vi "Read_Flow_Press_Bkgd_Mvg_avg.vi"() -> ()   [LabVIEW 2016]
uses:
  <userlib>/Fluigent/Fluigent MFCS/FluigentMFCS_Full.llb/MFCS_EZ Detect.vi
  <userlib>/Fluigent/Fluigent MFCS/FluigentMFCS_Full.llb/MFCS_EZ Initialization.vi
  Globals/PressuresGlobal.vi
  <vilib>/Analysis/baseanly.llb/Unimode.vi
  <vilib>/imath/engines/lvmath2/RunTimeEngine/BuiltInFunctions/size/NIMS_I32=size(GM,I32).vi
  <instcachedir>/0/NIMS_I32=size(GM,I32)_9B6975FE2A37478D9DF1A6A9597B9E6B.lvgen/NIMS_I32=size(GM,I32)_9B6975FE2A37478D9DF1A6A9597B9E6B_004.vi
  <vilib>/imath/engines/lvmath2/RunTimeEngine/BuiltInFunctions/zeros/NIMS_V=zeros(I32,I32).vi
  <vilib>/imath/engines/lvmath2/RunTimeEngine/ErrorHandling/NIMS_Create Error From Enums.vi
  <vilib>/imathl/engines/lvmath/Functions/Error Handling/Create Error.vi
  <vilib>/imath/engines/lvmath2/RunTimeEngine/RangeToken/NIMS_Range_R2 - Integer.vi
  <instcachedir>/0/NIMS_Range_R2 - Integer_416A044C4F024DBE8E97DA138CB3186F.lvgen/NIMS_Range_R2 - Integer_416A044C4F024DBE8E97DA138CB3186F_000.vi
  <vilib>/imath/engines/lvmath2/RunTimeEngine/CommandStatement/MC_CommandStatement_break.vi
  <vilib>/imath/engines/lvmath2/RunTimeEngine/IndexRead/NIMS M($,S).vi
  <instcachedir>/0/NIMS M($,S)_3E5749BBB62E49528D4765A77F1F6D98.lvgen/NIMS M($,S)_3E5749BBB62E49528D4765A77F1F6D98_000.vi
  <vilib>/imath/engines/lvmath2/RunTimeEngine/BuiltInFunctions/sets_unique/NIMS_sets_unique(GV).vi
  <instcachedir>/0/NIMS_sets_unique(GV)_BC60CBD939E647F382369330BF9EA64D.lvgen/NIMS_sets_unique(GV)_BC60CBD939E647F382369330BF9EA64D_001.vi
  <vilib>/imath/engines/lvmath2/RunTimeEngine/BuiltInFunctions/length/NIMS_length(GV).vi
  <instcachedir>/0/NIMS_length(GV)_08A3D13377FD4E4B96F5795FBF3698FA.lvgen/NIMS_length(GV)_08A3D13377FD4E4B96F5795FBF3698FA_000.vi
  <vilib>/imath/engines/lvmath2/RunTimeEngine/IndexReplace/NIMS V(S)=S.vi
  <instcachedir>/0/NIMS V(S)=S_5B9D821375184D3582A2146CD1A04ED7.lvgen/NIMS V(S)=S_5B9D821375184D3582A2146CD1A04ED7_003.vi
  <vilib>/imath/engines/lvmath2/RunTimeEngine/NodeEndStatement/NIMS_NodeEndStatement_Output.vi
  <instcachedir>/0/NIMS_NodeEndStatement_Output_53EC0D466D134D7ABD903AC30B43404B.lvgen/NIMS_NodeEndStatement_Output_53EC0D466D134D7ABD903AC30B43404B_004.vi
  <vilib>/imath/engines/lvmath2/RunTimeEngine/ErrorHandling/NIMS_Finalize Error.vi
  <userlib>/Fluigent/Fluigent MFCS/FluigentMFCS_Full.llb/MFCS_EZ Read All Channels Pressure.vi
  <vilib>/Analysis/NI_AALBase.lvlib
panel:
  in  "reset averaging":bool
  out "Pressure Stable?":bool=TRUE
  in  "reset volume":bool
  out "Volume":dbl[](array[numeric])
  out "Median":dbl[](array[numeric])
  out "Mode":dbl[](array[numeric])
  out "numUnique":i32[](array[numeric])
  out "sum":dbl
  out "pressure array":dbl[][](array[numeric])
  in  "Time to include":dbl=5.0
  out "dt(calc)":dbl
  out "freq (Hz)":dbl
  out "Sample Rate":dbl(graph)
  in  "stop":bool
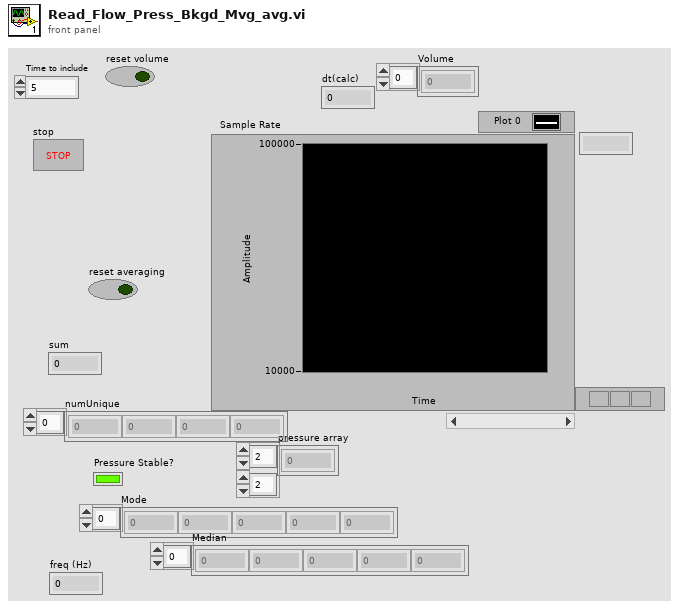
[diagram p1: front panel]
types:
  T1 = cluster{"Time":dbl, "All Flow-Rates":dbl[], "Flow 2 Filter Time":dbl, "Flow 1 Filter Time":dbl}
  T2 = typedef "_EZmfcsSN.ctl" = u16
  T3 = typedef "_EZmfcsRefNum.ctl" = refnum<k1>
  T4 = typedef "_frpRefNum" = refnum<k1>
  T5 = cluster{"relative seconds":dbl, "All Flow-Rates":dbl[], "Flow 1 Filter Time":dbl, "Flow 2 Filter Time":dbl}
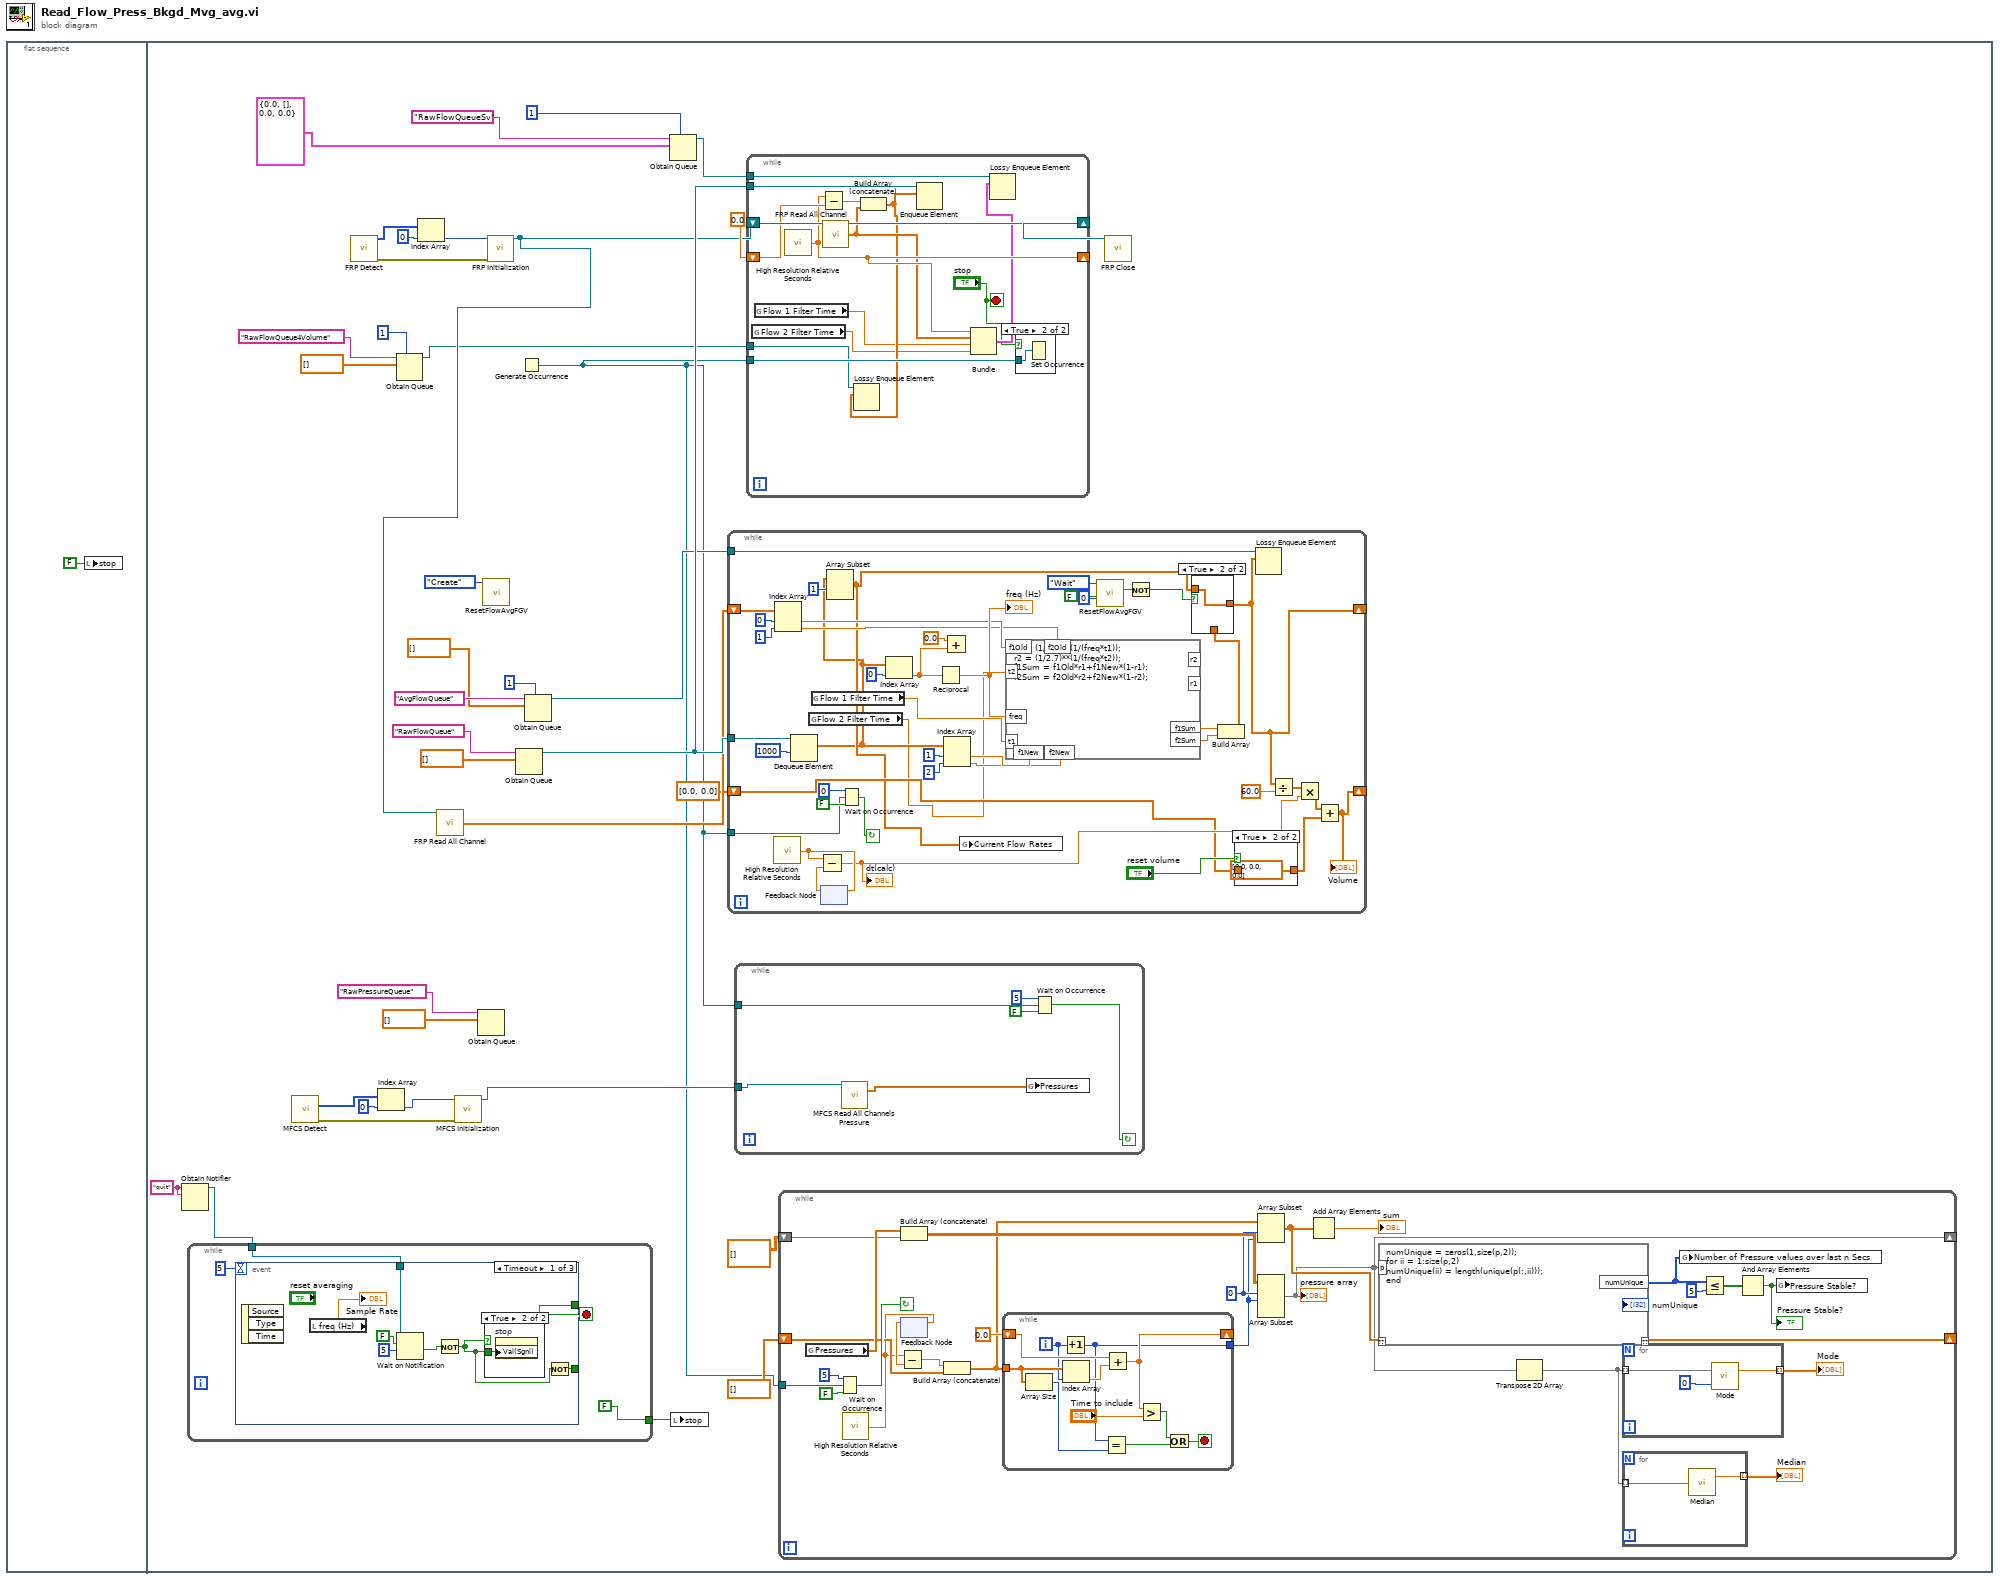
[diagram p0: block diagram]
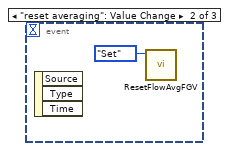
[diagram p5: hidden frame]
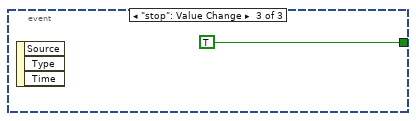
[diagram p6: hidden frame]
diagram:
  n1 = flat-sequence {
    frame #0 {
      n2 = local write "stop"(FALSE ("stop")) -> ()
    }
    frame #1 {
      w5 = "quit" ("name (unnamed)")
      n3 = Obtain Notifier(name (unnamed)=w5, notification data type=w5) -> (notifier out=w3:refnum<notifier>)  [unwired: 2 in, 2 out]
      n4 = while {
        tunnel: w3 -> [w247]
        tunnel: [FALSE] -> w2
        stop <- w248 stop-if-true
        n5 = event shown="[0] Timeout" {
          selector: _ -> [_ _ _]
          dyn-events: _ -> [_ _ _]
          timeout: 5 -> [_ _ _]
          tunnel: [_ _ TRUE] -> w248
          tunnel: w247 -> [w252 _ _]
          tunnel: [w250 _ _] -> _
          event Timeout {
            n6 = event-data() -> ()  [unwired: 1 in, 3 out]
            n7 = local read "freq (Hz)"() -> (→"Sample Rate":dbl)
            n8 = Wait on Notification(notifier=w252, ignore previous (F)=FALSE, timeout in ms (-1)=5) -> (timed out?=w254:bool)  [unwired: 1 in, 3 out]
            n9 = Not(x=w254) -> (.not. x?=w251:bool)
            n10 = case shown="True" w251 {
              tunnel: w251 -> [_ w257]
              frame False {
              }
              frame True {
                n11 = property on="stop" class="Bool (strict)"("Val(Sgnl)"=w257) -> ()  [unwired: 2 in, 2 out]
              }
            }
            n12 = Not(x=w251) -> (.not. x?=w250:bool)
          }
          event "reset averaging": Value Change {
            n13 = event-data() -> ()  [unwired: 1 in, 3 out]
            n14 = call "ResetFlowAvgFGV.vi"("Action"=enum16{"Create", "Set", "Wait"}."Set") -> ()  [unwired: 10 in, 1 out]
          }
          event "stop": Value Change {
            n15 = event-data() -> ()  [unwired: 1 in, 3 out]
          }
        }
      }
      n16 = call-poly <userlib>:"MFCS Detect.vi"() -> ("[SN MFCS_EZ]"=w15:T2[], "error out"=w17:errorcluster)  [unwired: 14 in]
      n17 = call <userlib>:"FRP Detect.vi"() -> ("FLOWBOARD List"=w39:u16[], "error out"=w37:errorcluster)  [unwired: 14 in]
      n18 = Index Array(array=w15, index=0) -> (element=w16:T2)
      n19 = Obtain Queue(max queue size (-1, unlimited)=1, name (unnamed)="RawFlowQueue4Volume", element data type=dbl[] [] ("appended array")) -> (queue out=w7:refnum<queue>)  [unwired: 2 in, 2 out]
      n20 = Index Array(array=w39, index=0) -> (element=w36:u16)
      n21 = call-poly <userlib>:"MFCS Initialization.vi"("SN MFCS_EZ"=w16, "error in (no error)"=w17) -> ("MFCS_EZ"=w14:T3)  [unwired: 11 in, 2 out]
      n22 = Obtain Queue(name (unnamed)="RawPressureQueue", element data type=dbl[] [] ("appended array")) -> ()  [unwired: 3 in, 3 out]
      n23 = call "ResetFlowAvgFGV.vi"("Action"=enum16{"Create", "Set", "Wait"}."Create") -> ()  [unwired: 10 in, 1 out]
      n24 = call <userlib>:"FRP Initialization.vi"("Serial Number"=w36, "error in (no error)"=w37) -> ("FRP out"=w28:T4)  [unwired: 11 in, 2 out]
      n25 = call <userlib>:"FRP Read All Channel.vi"("FRP"=w28) -> ("All Flow-Rates"=w27:dbl[])  [unwired: 12 in, 2 out]
      n26 = Obtain Queue(name (unnamed)="RawFlowQueue", element data type=dbl[] [] ("appended array")) -> (queue out=w31:refnum<queue>)  [unwired: 3 in, 2 out]
      n27 = Generate Occurrence() -> (w4:refnum<k4>)
      n28 = Obtain Queue(max queue size (-1, unlimited)=1, name (unnamed)="AvgFlowQueue", element data type=dbl[] [] ("appended array")) -> (queue out=w25:refnum<queue>)  [unwired: 2 in, 2 out]
      n29 = Obtain Queue(max queue size (-1, unlimited)=1, name (unnamed)="RawFlowQueueSv", element data type=T1 {"Time"=0.0, "All Flow-Rates"=[], "Flow 2 Filter Time"=0.0, "Flow 1 Filter Time"=0.0} ("output cluster")) -> (queue out=w23:refnum<queue>)  [unwired: 2 in, 2 out]
      n30 = local write "stop"(w2) -> ()
      n31 = while {
        tunnel: w31 -> [w241]
        tunnel: w25 -> [w239]
        shift-right: [w204] -> _
        shift-left: w27 -> [w218]
        tunnel: w4 -> [w220]
        shift-right: [w210] -> _
        shift-left: dbl[] [0.0, 0.0] -> [w212]
        stop <- w219 continue-if-true
        n32 = call <vilib>:"High Resolution Relative Seconds.vi"() -> ("relative seconds"=w223:dbl)
        n33 = Index Array(array=w218, index #1=0 ("index"), index #2=1 ("index")) -> (element #1=w230:dbl, element #2=w229:dbl)
        n34 = Dequeue Element(queue=w241, timeout in ms (-1)=1000) -> (element=w200:dbl[])  [unwired: 1 in, 3 out]
        n35 = global read "PressuresGlobal.vi" "Flow 2 Filter Time"() -> (w198:dbl)
        n36 = global read "PressuresGlobal.vi" "Flow 1 Filter Time"() -> (w199:dbl)
        n37 = feedback-in #1(w223) -> ()
        n38 = feedback #1() -> (w224:dbl)  [unwired: 1 in]
        n39 = Subtract(x=w223, y=w224) -> (x-y=w215:dbl)
        "dt(calc)" <- w215
        n40 = Array Subset(array=w200, index=1) -> (w201:dbl[])  [unwired: 1 in]
        n41 = Wait on Occurrence(1:FALSE ("ignore previous (T)"), 2:w220, 3:0 ("ms timeout (-1)")) -> (0:w219:bool)
        n42 = Index Array(array=w200, index=0) -> (element=w235:dbl)
        n43 = Reciprocal(x=w235) -> (1/x=w234:dbl)
        "freq (Hz)" <- w234
        n44 = Add(x=0.0 ("Flow-Rate"), y=w235) -> ()  [unwired: 1 out]
        n45 = Index Array(array=w200, index #1=1 ("index"), index #2=2 ("index")) -> (element #1=w228:dbl, element #2=w227:dbl)
        n46 = global write "PressuresGlobal.vi" "Current Flow Rates"(w201) -> ()
        n47 = formula code="r1 = (1/2.7)**(1/(freq*t1));\nr2 = (1/2.7)**(1/(freq*t2));\nf1Sum = f1Old*r1+f1New*(1-r1);\nf2Sum = f2Old*r2+f2New*(1-r2);"("freq"=w234, "t1"=w199, "t2"=w198, "f1Old"=w230, "f2Old"=w229, "f1New"=w228, "f2New"=w227) -> ("f1Sum"=w225:dbl, "f2Sum"=w226:dbl)  [unwired: 2 out]
        n48 = call "ResetFlowAvgFGV.vi"("ignore previous (T)"=FALSE, "timeout in ms (-1)"=0, "Action"=enum16{"Create", "Set", "Wait"}."Wait") -> ("timed out?"=w206:bool)  [unwired: 8 in]
        n49 = Not(x=w206) -> (.not. x?=w205:bool)
        n50 = Build Array(w225, w226) -> (w203:dbl[])
        n51 = case shown="True" w205 {
          tunnel: w201 -> [_ w243]
          tunnel: [w242 w243] -> w204
          tunnel: w203 -> [w242 _]
          frame False {
          }
          frame True {
          }
        }
        n52 = case shown="True" "reset volume" {
          tunnel: w212 -> [w244 _]
          tunnel: [w244 dbl[] [0.0, 0.0, 0.0]] -> w211
          frame False {
          }
          frame True {
          }
        }
        n53 = Lossy Enqueue Element(queue=w239, element=w204) -> ()  [unwired: 1 in, 4 out]
        n54 = Divide(x=w204, y=60.0) -> (x/y=w216:dbl[])
        n55 = Multiply(x=w216, y=w215) -> (x*y=w214:dbl[])
        n56 = Add(x=w214, y=w211) -> (x+y=w210:dbl[])
        "Volume" <- w210
      }
      n57 = while {
        tunnel: w14 -> [w197]
        tunnel: w4 -> [w195]
        stop <- w192 continue-if-true
        n58 = call-poly <userlib>:"MFCS Read All Channels Pressure.vi"("MFCS_EZ"=w197) -> ("All Channels Pressure"=w196:dbl[])  [unwired: 12 in, 2 out]
        n59 = global write "PressuresGlobal.vi" "Pressures"(w196) -> ()
        n60 = Wait on Occurrence(1:FALSE ("ignore previous (T)"), 2:w195, 3:5 ("ms timeout (-1)")) -> (0:w192:bool)
      }
      n61 = while {
        shift-right: [w273] -> w35
        shift-left: w28 -> [w274]
        shift-right: [w268] -> _
        shift-left: 0.0 ("relative seconds") -> [w272]
        tunnel: w31 -> [w270]
        tunnel: w23 -> [w269]
        tunnel: w4 -> [w265]
        tunnel: w7 -> [w264]
        stop <- "stop" stop-if-true
        n62 = global read "PressuresGlobal.vi" "Flow 2 Filter Time"() -> (w261:dbl)
        n63 = global read "PressuresGlobal.vi" "Flow 1 Filter Time"() -> (w262:dbl)
        n64 = call <vilib>:"High Resolution Relative Seconds.vi"() -> ("relative seconds"=w268:dbl)
        n65 = Subtract(x=w268, y=w272) -> (x-y=w271:dbl)
        n66 = call <userlib>:"FRP Read All Channel.vi"("FRP"=w274) -> ("FRP out"=w273:T4, "All Flow-Rates"=w267:dbl[])  [unwired: 12 in, 1 out]
        n67 = Build Array (concatenate)(w271, w267) -> (w263:dbl[])
        n68 = Lossy Enqueue Element(queue=w264, element=w263) -> ()  [unwired: 1 in, 4 out]
        n69 = Enqueue Element(queue=w270, element=w263) -> ()  [unwired: 2 in, 3 out]
        n70 = Bundle("relative seconds"=w268, "All Flow-Rates"=w267, "Flow 1 Filter Time"=w262, "Flow 2 Filter Time"=w261) -> (w266:T5)  [unwired: 1 in]
        n71 = Lossy Enqueue Element(queue=w269, element=w266) -> ()  [unwired: 1 in, 4 out]
        n72 = case shown="True" "stop" {
          tunnel: w265 -> [_ w275]
          frame False {
          }
          frame True {
            n73 = Set Occurrence(w275) -> ()
          }
        }
      }
      n74 = while {
        tunnel: w4 -> [w61]
        shift-right: [w47] -> _
        shift-left: dbl[][] [] -> [w56]
        shift-right: [w51] -> _
        shift-left: dbl[] [] -> [w55]
        stop <- w62 continue-if-true
        w53 = 0 ("index")
        n75 = global read "PressuresGlobal.vi" "Pressures"() -> (w59:dbl[])
        n76 = Wait on Occurrence(1:FALSE ("ignore previous (T)"), 2:w61, 3:5 ("ms timeout (-1)")) -> (0:w62:bool)
        n77 = call <vilib>:"High Resolution Relative Seconds.vi"() -> ("relative seconds"=w49:dbl)
        n78 = Build Array (concatenate)(w59, w56) -> (w57:dbl[][])
        n79 = feedback #2() -> (w60:dbl)  [unwired: 1 in]
        n80 = Subtract(x=w49, y=w60) -> (x-y=w48:dbl)
        n81 = feedback-in #2(w49) -> ()
        n82 = Build Array (concatenate)(w48, w55) -> (w54:dbl[])
        n83 = while {
          tunnel: w54 -> [w187]
          shift-right: [w189] -> _
          shift-left: 0.0 ("relative seconds") -> [w191]
          tunnel: [w181] -> w52
          i -> [w182]
          stop <- w183 stop-if-true
          n84 = Array Size(array=w187) -> (size(s)=w186:i32)
          n85 = Increment(x=w182) -> (x+1=w181:i32)
          n86 = Index Array(array=w187, index=w182) -> (element=w190:dbl)
          n87 = Equal?(x=w181, y=w186) -> (x = y?=w185:bool)
          n88 = Add(x=w191, y=w190) -> (x+y=w189:dbl)
          n89 = Greater?(x=w189, y="Time to include") -> (0:w184:bool)
          n90 = Or(x=w184, y=w185) -> (x .or. y?=w183:bool)
        }
        n91 = Array Subset(array=w54, index=w53, length=w52) -> (w51:dbl[])
        n92 = Array Subset(array=w57, index (row)=w53, length (row)=w52) -> (w47:dbl[][])  [unwired: 2 in]
        "pressure array" <- w47
        n93 = Add Array Elements(numeric array=w51) -> (sum=→"sum":dbl)
        n94 = mathscript code="numUnique = zeros(1,size(p,2));\nfor ii = 1:size(p,2)\nnumUnique(ii) = length(unique(p(:,ii)));\nend"("p"=w47) -> ("numUnique"=w40:i32[])  [unwired: 1 in, 1 out]
        "numUnique" <- w40
        n95 = Transpose 2D Array(2D array=w47) -> (transposed array=w45:dbl[][])
        n96 = for {
          tunnel: w45 -> [w69] mode=indexing
          tunnel: [w68] -> w46 mode=indexing
          n97 = call-poly <vilib>:"Mode.vi"("intervals"=0, "X"=w69) -> ("mode"=w68:dbl)  [unwired: 1 out]
        }
        "Mode" <- w46
        n98 = for {
          tunnel: w45 -> [w66] mode=indexing
          tunnel: [w65] -> w44 mode=indexing
          n99 = call <vilib>:"Median.vi"("X"=w66) -> ("median"=w65:dbl)  [unwired: 1 out]
        }
        "Median" <- w44
        n100 = global write "PressuresGlobal.vi" "Number of Pressure values over last n Secs"(w40) -> ()
        n101 = Less Or Equal?(x=w40, y=5) -> (x <= y?=w42:bool[])
        n102 = And Array Elements(Boolean array=w42) -> (logical AND=w41:bool)
        "Pressure Stable?" <- w41
        n103 = global write "PressuresGlobal.vi" "Pressure Stable?"(w41) -> ()
      }
      n104 = call <userlib>:"FRP Close.vi"("FRP"=w35) -> ()  [unwired: 14 in, 1 out]
    }
  }
